vi "Shoot Global.vi"() -> ()   [LabVIEW 2019]
uses:
  Shooter Command Type Def.ctl
  Shooter Mode Type Def.ctl
  Shooter Preset speeds Type Def.ctl
  Calculations or utilities/Is command done typedef.ctl
panel:
  out "Shooter Command Done?":T1
  in  "Shoot Auton Command":T2={"Shooter Mode"=enum."Disabled", "Throttle (%)/ Vision-based\nSetpoint (RPM)"=0.0, "Shooter Preset speeds (RPM)"=enum."Target Zone", "Timestamp (ms)"=0.0}
  in  "Shoot Teleop Command":T2={"Shooter Mode"=enum."Disabled", "Throttle (%)/ Vision-based\nSetpoint (RPM)"=0.0, "Shooter Preset speeds (RPM)"=enum."Target Zone", "Timestamp (ms)"=0.0}
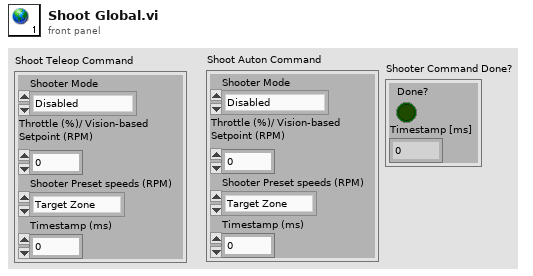
[diagram p1: front panel]
types:
  T1 = typedef "Is command done typedef.ctl" = cluster{"Done?":bool, "Timestamp [ms]":dbl}
  T2 = typedef "Shooter Command Type Def.ctl" = cluster{"Shooter Mode":T3, "Throttle (%)/ Vision-based\nSetpoint (RPM)":dbl, "Shooter Preset speeds (RPM)":T4, "Timestamp (ms)":dbl}
  T3 = typedef "Shooter Mode Type Def.ctl" = enum16{"Disabled", "Raw Throttle", "Preset Velocity Control", "Vision-based Velocity Control"}
  T4 = typedef "Shooter Preset speeds Type Def.ctl" = enum16{"Not Applicable", "Target Zone", "Initiation Line", "Close end of Trench Run", "Control Panel"}
diagram:
